vi "checkIsVI.vi"(8 "error in (no error)":errorcluster, 10 "Name":string, 11 "VI in":refnum<class "VI.lvclass">) -> (0 "error out":errorcluster, 2 "isVI?":bool, 3 "VI out":refnum<class "VI.lvclass">)   [LabVIEW 2016, in "VI.lvclass"]
uses:
  VI.lvclass
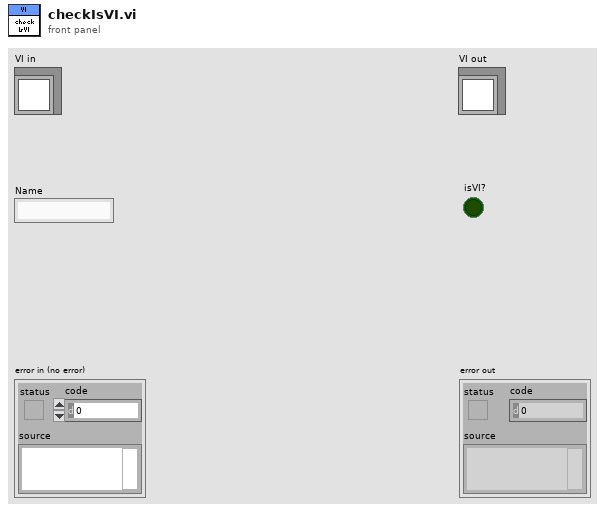
[diagram p1: front panel]
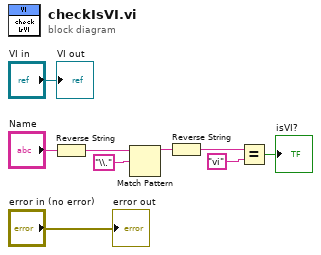
[diagram p0: block diagram]
diagram:
  n1 = Reverse String(1:"Name") -> (0:w6:string)
  n2 = Match Pattern(string=w6, regular expression="\\.") -> (before substring=w5:string)  [unwired: 1 in, 3 out]
  n3 = Reverse String(1:w5) -> (0:w3:string)
  n4 = Equal?(x=w3, y="vi") -> (x = y?=→"isVI?":bool)
  "error out" <- "error in (no error)"
  "VI out" <- "VI in"
